vi "Get library version.vi"(8 "error in (no error)":errorcluster, 9 "library name in":string=".lvlib", 10 "Top Level/Always Included VIs":path[](array[path]), 11 "Target reference in":refnum<vi>) -> (0 "error out":errorcluster, 1 "Library Found":bool, 2 "Version":T1, 3 "Target reference out":refnum<vi>, 5 "found library name":string)   [LabVIEW 2021, in "CIF Build Actions.lvlib"]
uses:
  CIF Build Actions.lvlib
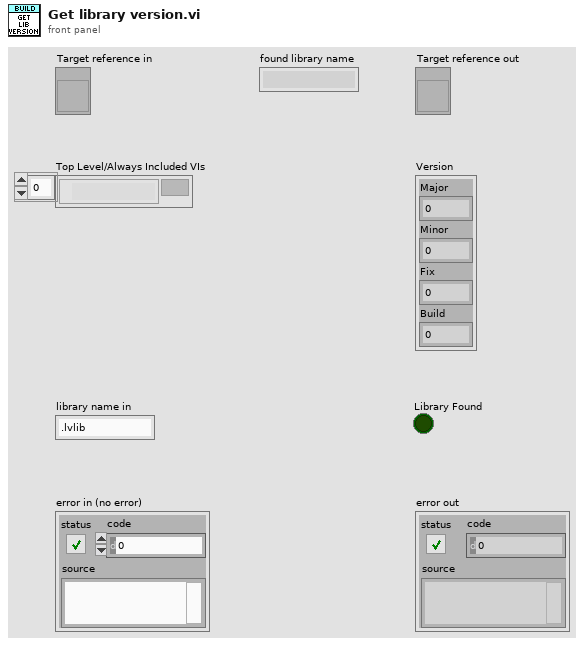
[diagram p1: front panel]
types:
  T1 = cluster{"Major":u16, "Minor":u16, "Fix":u16, "Build":u16}
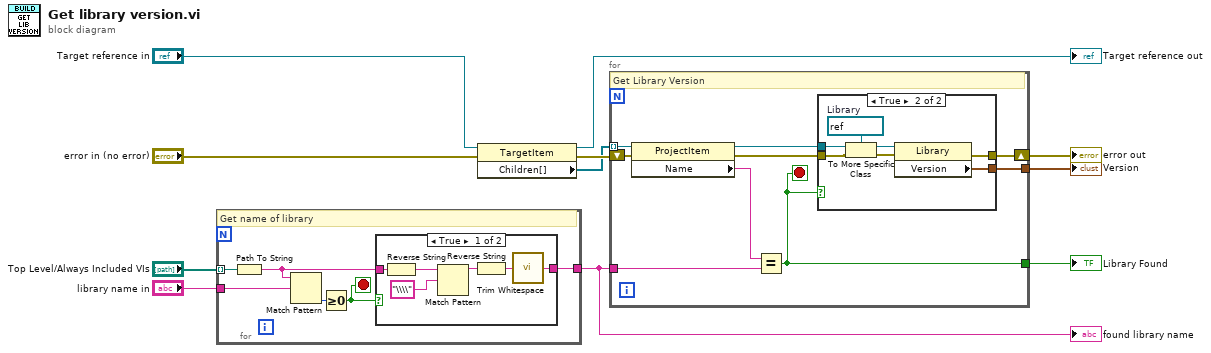
[diagram p0: block diagram]
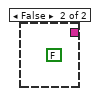
[diagram p2: hidden frame]
diagram:
  n1 = for {
    tunnel: "Top Level/Always Included VIs" -> [w17] mode=indexing
    tunnel: [w14] -> w5
    tunnel: "library name in" -> [w12]
    stop <- w13 stop-if-true
    # "Get name of library"
    n2 = Path To String(path=w17) -> (string=w15:string)
    n3 = Match Pattern(string=w15, regular expression=w12) -> (offset past match=w16:i32)  [unwired: 1 in, 3 out]
    n4 = Greater Or Equal To 0?(x=w16) -> (x >= 0?=w13:bool)
    n5 = case shown="True" w13 {
      tunnel: w15 -> [w23 _]
      tunnel: [w18 _] -> w14
      frame True {
        n6 = Reverse String(1:w23) -> (0:w20:string)
        n7 = Match Pattern(string=w20, regular expression="\\\\") -> (before substring=w21:string)  [unwired: 1 in, 3 out]
        n8 = Reverse String(1:w21) -> (0:w19:string)
        n9 = call <vilib>:"Trim Whitespace.vi"("string"=w19) -> ("trimmed string"=w18:string)  [unwired: 1 in]
      }
      frame False {
        (unwired) FALSE
      }
    }
  }
  "found library name" <- w5
  n10 = property class="TargetItem"(reference="Target reference in", error in="error in (no error)") -> (reference out=→"Target reference out":refnum<vi>, error out=w6:errorcluster, "Children[]"=w2:refnum<vi>[])
  n11 = for {
    tunnel: w2 -> [w31] mode=indexing
    tunnel: [w32] -> w10
    tunnel: w5 -> [w30]
    tunnel: [w28] -> w1
    shift-right: [w26] -> w11
    shift-left: w6 -> [w25]
    stop <- w28 stop-if-true
    # "Get Library Version"
    n12 = property class="ProjectItem"(reference=w31, error in=w25) -> (reference out=w29:refnum<vi>, error out=w27:errorcluster, "Name"=w24:string)
    n13 = Equal?(x=w24, y=w30) -> (x = y?=w28:bool)
    n14 = case shown="True" w28 {
      tunnel: [_ w38] -> w32
      tunnel: w29 -> [_ w37]
      tunnel: w27 -> [w33 w36]
      tunnel: [w33 w34] -> w26
      frame False {
      }
      frame True {
        w39 = refnum<vi> refnum  # Library
        n15 = To More Specific Class(target class=w39, reference=w37, error in=w36) -> (specific class reference=w40:refnum<vi>, error out=w35:errorcluster)
        n16 = property class="Library"(reference=w40, error in=w35) -> (error out=w34:errorcluster, "Version"=w38:T1)  [unwired: 1 out]
      }
    }
  }
  "error out" <- w11
  "Version" <- w10
  "Library Found" <- w1
